vi "EIP channel to string.vi"(11 "channel in":refnum<class "EIP Tags Channel.lvclass">) -> (2 "channel data":string, 3 "identifier":string)   [LabVIEW 2013, in "EIP Tags Channel.lvclass"]
uses:
  EIP Tags Channel.lvclass
  <vilib>/NI/Tag Bus/tag/tag descriptor.lvclass/tag descriptor.ctl
  <vilib>/NI/Tag Bus Module Framework/channel/TBM channel.lvclass/TBM channel.ctl
  EIP Tags Channel.lvclass/EIP Tags Channel.ctl
  <vilib>/NI/Tag Bus/tag/tag descriptor.lvclass
  <vilib>/NI/Tag Bus Module Framework/channel/TBM channel.lvclass
  <vilib>/NI/Configuration Framework/serializable configuration/NISE_CEF_serializable configuration.lvclass
panel:
  out "error out":errorcluster
  in  "error in":errorcluster
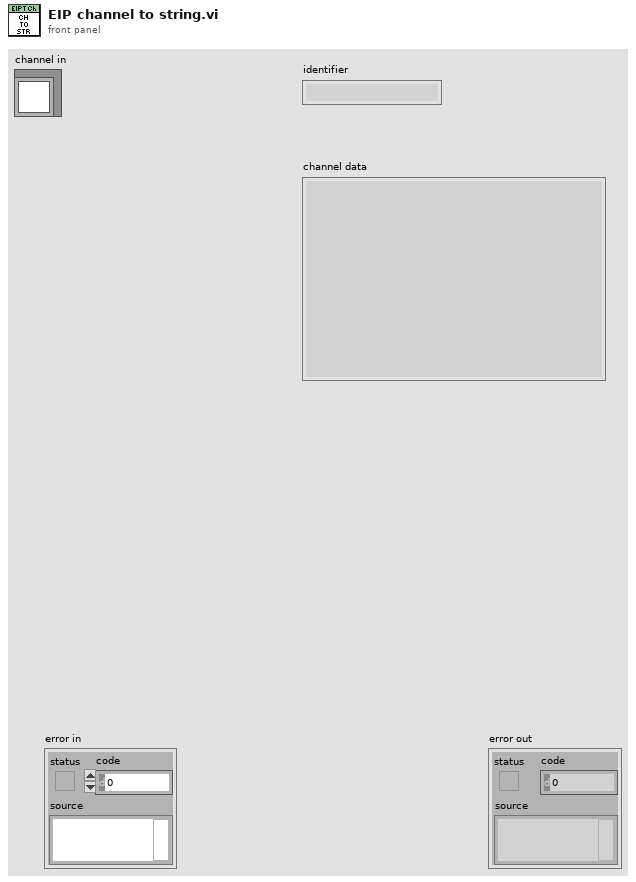
[diagram p1: front panel]
types:
  T1 = typedef "tag bus.lvlib/tag descriptor.lvclass/Data Type.ctl" = enum16{"Double", "Single", "I64", "I32", "I16", "I8", "U64", "U32", "U16", "U8", "Boolean", "String", "Array of Double", "Array of Single", "Array of I64", "Array of I32", "Array of I16", "Array of I8", "Array of U64", "Array of U32", "Array of U16", "Array of U8", "Array of Boolean", "Array of String"}
  T2 = typedef "TBM channel.lvclass/channel classification.ctl" = enum16{"input data", "output data", "processing parameter", "processing result"}
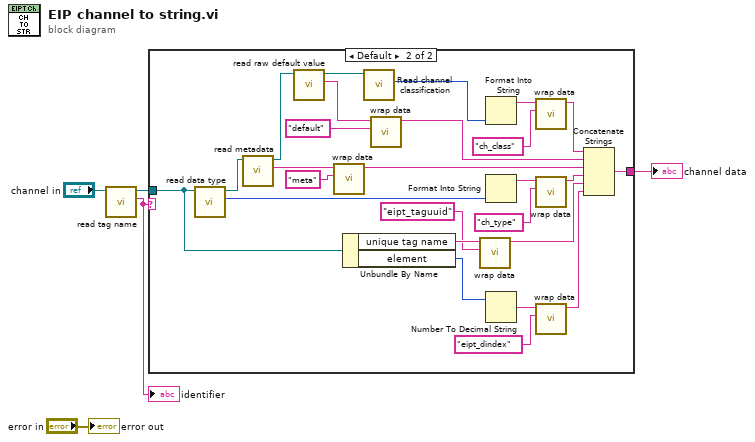
[diagram p0: block diagram]
diagram:
  n1 = call <vilib>:"read tag name.vi"("system tag in"="channel in") -> ("name"=w2:string, "system tag out"=w3:refnum<class "EIP Tags Channel.lvclass">)  [unwired: 8 in, 1 out]
  "identifier" <- w2
  n2 = case shown="Default" w2 {
    selector: w2 -> [w6 _]
    tunnel: [w6 w15] -> w5
    tunnel: w3 -> [_ w14]
    frame "" {
    }
    frame Default {
      n3 = call <vilib>:"read data type.vi"("system tag in"=w14) -> ("data type"=w30:T1, "system tag out"=w32:refnum<class "EIP Tags Channel.lvclass">)  [unwired: 8 in, 1 out]
      n4 = call <vilib>:"read metadata.vi"("system tag in"=w32) -> ("metadata"=w25:string, "system tag out"=w31:refnum<class "EIP Tags Channel.lvclass">)  [unwired: 8 in, 1 out]
      n5 = call <vilib>:"read raw default value.vi"("system tag in"=w31) -> ("raw default"=w24:string, "system tag out"=w27:refnum<class "EIP Tags Channel.lvclass">)  [unwired: 8 in, 1 out]
      n6 = call <vilib>:"wrap data.vi"("identifier"="meta", "data to wrap"=w25) -> ("wrapped data"=w17:string)  [unwired: 9 in]
      n7 = Unbundle By Name(w14) -> ("unique tag name"=w13:string, "element"=w12:i32)
      n8 = call <vilib>:"Read channel classification.vi"("channel in"=w27) -> ("channel classification"=w22:T2)  [unwired: 8 in, 2 out]
      n9 = call <vilib>:"wrap data.vi"("identifier"="default", "data to wrap"=w24) -> ("wrapped data"=w18:string)  [unwired: 9 in]
      n10 = call <vilib>:"wrap data.vi"("identifier"="eipt_taguuid", "data to wrap"=w13) -> ("wrapped data"=w7:string)  [unwired: 9 in]
      n11 = Format Into String(w22) -> (resulting string=w21:string)  [unwired: 3 in, 1 out]
      n12 = Format Into String(w30) -> (resulting string=w29:string)  [unwired: 3 in, 1 out]
      n13 = Number To Decimal String(number=w12) -> (decimal integer string=w9:string)  [unwired: 1 in]
      n14 = call <vilib>:"wrap data.vi"("identifier"="ch_class", "data to wrap"=w21) -> ("wrapped data"=w19:string)  [unwired: 9 in]
      n15 = call <vilib>:"wrap data.vi"("identifier"="ch_type", "data to wrap"=w29) -> ("wrapped data"=w16:string)  [unwired: 9 in]
      n16 = call <vilib>:"wrap data.vi"("identifier"="eipt_dindex", "data to wrap"=w9) -> ("wrapped data"=w8:string)  [unwired: 9 in]
      n17 = Concatenate Strings(w19, w18, w17, w16, w7, w8) -> (w15:string)
    }
  }
  "channel data" <- w5
  "error out" <- "error in"
